vi "Wait For Compile.vi"(11 "target in":refnum<class "Base Target.lvclass">) -> (0 "compiled":bool, 3 "target out":refnum<class "Base Target.lvclass">)   [LabVIEW 2020, in "NI_TargetHelper.lvlib" / "Base Target.lvclass"]
uses:
  <vilib>/TargetSupport/NI_TargetHelper/Base Target/Base Target.lvclass
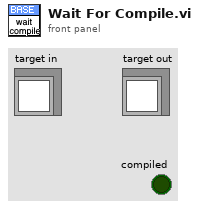
[diagram p1: front panel]
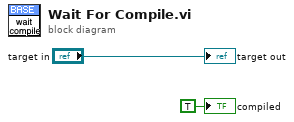
[diagram p0: block diagram]
diagram:
  "target out" <- "target in"
  "compiled" <- TRUE ("compiled")
